vi "Read AngularConfig.vi"(8 "error in (no error)":errorcluster, 11 "Angular_Task in":refnum<class "Angular_Task.lvclass">) -> (0 "error out":errorcluster, 2 "AngularConfig":T2(c390), 3 "Angular_Task out":refnum<class "Angular_Task.lvclass">)   [LabVIEW 2025, in "Angular_Task.lvlib" / "Angular_Task.lvclass"]
uses:
  Angular_Task.lvclass
  Angular_Task.lvclass/Angular_Task.ctl
  DAQ_Module/DAQ_Module/DAQ_Module/DAQ_Angular_Task_Config.ctl
  DAQ_Module/DAQ_Module/DAQ_Module/DAQ_Module.lvclass
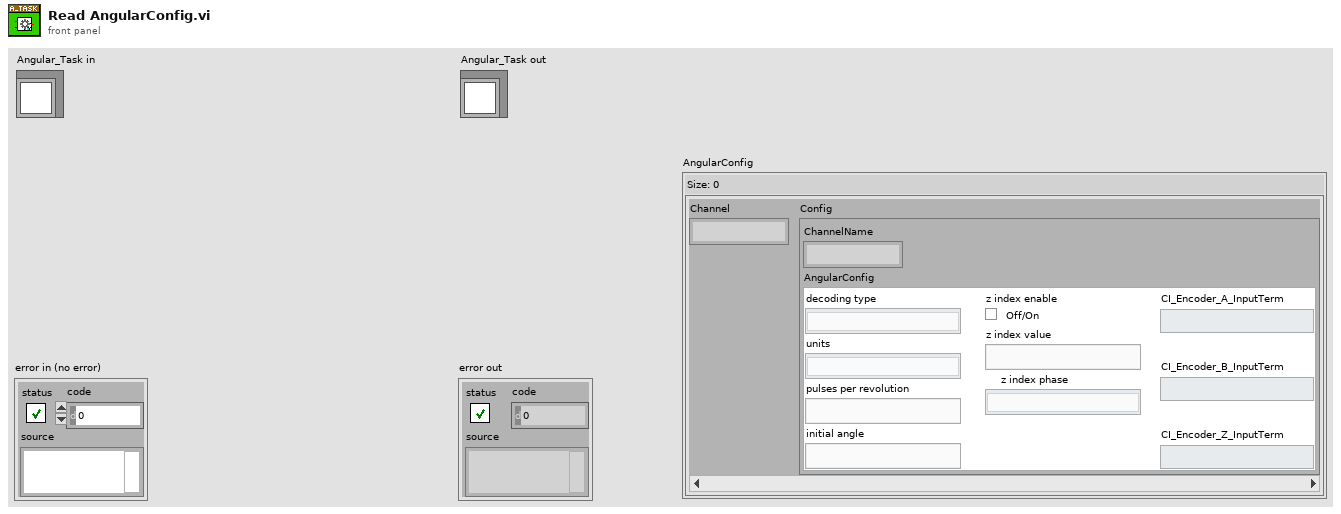
[diagram p1: front panel]
types:
  T1 = typedef "DAQ_Module.lvlib/DAQ_Module.lvclass/DAQ_Angular_Task_Config.ctl" = cluster{"decoding type":i32, "units":i32, "pulses per revolution":u32, "initial angle":dbl, "z index enable":bool, "z index value":dbl, "z index phase":i32, "CI_Encoder_A_InputTerm":string, "CI_Encoder_B_InputTerm":string, "CI_Encoder_Z_InputTerm":string}
  T2 = map{string, cluster{"ChannelName":string, "AngularConfig":T1}}
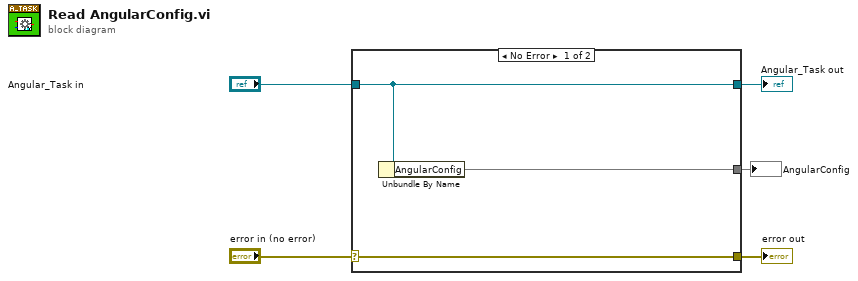
[diagram p0: block diagram]
diagram:
  n1 = case shown="No Error" "error in (no error)" {
    selector: "error in (no error)" -> [w8 w9]
    tunnel: [w8 w9] -> w4
    tunnel: [w7 w10] -> w2
    tunnel: "Angular_Task in" -> [w7 w10]
    tunnel: [w6 _] -> w1
    frame No Error {
      n2 = Unbundle By Name(w7) -> ("AngularConfig"=w6:T2)
    }
    frame Error {
    }
  }
  "error out" <- w4
  "Angular_Task out" <- w2
  "AngularConfig" <- w1
